vi "message_send.vi"(0 "Host_Reference":refnum<class "HGF_Reference.lvclass">, 1 "addressee":string, 2 "addressee interface":string, 3 "type":enum16{"mobile Agent", "Visitor", "Message"}(ring)=enum."Message", 4 "message":string, 5 "error in (no error)":errorcluster, 6 "request reply":bool=TRUE, 7 "message name":enum16{"travel request", "PublicKey"}(ring), 8 "timeout in ms (-1)":i32=-1, 9 "Object":refnum<class>, 11 "communication type":enum16{"SV", "Dim"}(ring)) -> (14 "dup Host_Reference":refnum<class "HGF_Reference.lvclass">, 19 "error out":errorcluster)   [LabVIEW 2009, in "MoAgSy.lvlib" / "MoAgSy_Host.lvclass"]
doc: "<B>Public</B> VI creates a new message and delivers it to addressee.\nReferenced Host is sender and will receive the reply.\n<B>still in progress\nError handling\n</B>\nF.Berck@gsi.de\nGSI Darmstadt 2009"
uses:
  MoAgSy_Host.lvclass
  HGF_BaseClasses/HGF_Reference/HGF_Reference.lvclass
  MoAgSy_Message/MoAgSy_Message.lvclass
  MoAgSy_Factory/MoAgSy_Factory.lvclass
  HGF_BaseClasses/HGF_Factory/HGF_Factory.lvclass
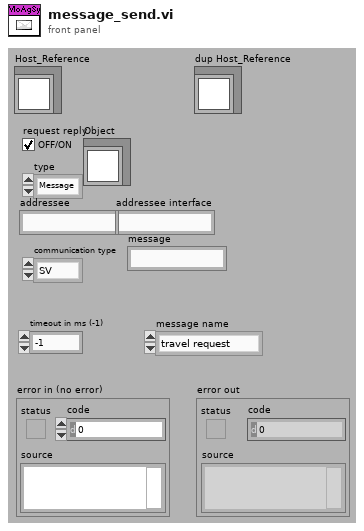
[diagram p1: front panel]
types:
  T1 = cluster{"Host Variable":refnum<k21>, "Agent_Event (Monitor Event)":refnum<class "HGF_Event.lvclass">, "Host_Event (Monitor Event)":refnum<class "HGF_Event.lvclass">, "DSCException":refnum<class "HGF_TriggeredEvent.lvclass">, "MoAgSy_DSCThreadPool":refnum<class "HGF_Reference.lvclass">, "ManagerEvent":refnum<class "HGF_Event.lvclass">, "DSCDestination":refnum<class "HGF_TriggeredEvent.lvclass">}
  T2 = cluster{"Host Name":string, "Maximum number of running Agents":i16, "ID":string}
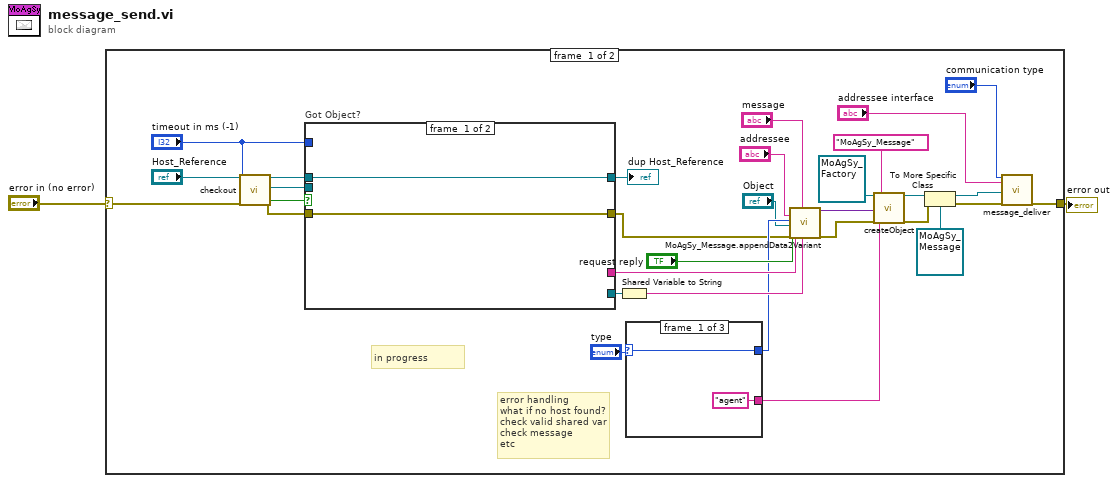
[diagram p0: block diagram]
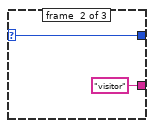
[diagram p2: hidden frame]
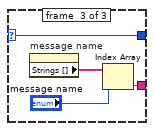
[diagram p3: hidden frame]
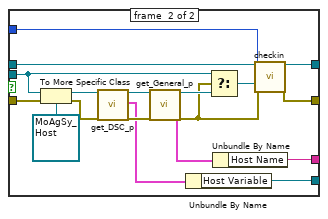
[diagram p4: hidden frame]
diagram:
  n1 = case shown="No Error" "error in (no error)" {
    selector: "error in (no error)" -> [w12 w62]
    tunnel: [w13 w62] -> w2
    frame #0 {
      # "error handling\nwhat if no host found?\ncheck valid shared var\ncheck message\netc"
      # "in progress"
      n2 = call "checkout.vi"("HGF_Reference"="Host_Reference", "timeout in ms (-1)"="timeout in ms (-1)", "error in (no error)"=w12) -> ("dup HGF_Reference"=w30:refnum<class "HGF_Reference.lvclass">, "Object"=w32:refnum<class>, "got object?"=w31:bool, "error out"=w33:errorcluster)  [unwired: 13 out]
      n3 = case "Got Object?" shown="True" w31 {
        tunnel: w32 -> [_ w54]
        tunnel: w30 -> [w43 w60]
        tunnel: [w43 w59] -> w28
        tunnel: "timeout in ms (-1)" -> [_ w58]
        tunnel: [w42 w57] -> w5
        tunnel: w33 -> [w42 w56]
        tunnel: [_ w50] -> w24
        tunnel: [_ w44] -> w15
        frame #0 {
        }
        frame #1 {
          n4 = To More Specific Class(target class=refnum<class "MoAgSy_Host.lvclass"> refnum ("MoAgSy.lvlib:MoAgSy_Host.lvclass"), reference=w54, error in=w56) -> (specific class reference=w49:refnum<class "MoAgSy_Host.lvclass">, error out=w47:errorcluster)
          n5 = call "get_DSC_p.vi"("MoAgSy_Host"=w49, "error in (no error)"=w47) -> ("dup MoAgSy_Host"=w48:refnum<class "MoAgSy_Host.lvclass">, "DSC"=w45:T1, "error out"=w46:errorcluster)  [unwired: 15 out]
          n6 = call "get_General_p.vi"("MoAgSy_Host"=w48, "error in (no error)"=w46) -> ("dup MoAgSy_Host"=w53:refnum<class "MoAgSy_Host.lvclass">, "General"=w51:T2, "error out"=w52:errorcluster)  [unwired: 15 out]
          n7 = Unbundle By Name(w45) -> ("Host Variable"=w44:refnum<k21>)
          n8 = Select(t=w54, s=w52, f=w53) -> (s? t:f=w55:refnum<class>)
          n9 = Unbundle By Name(w51) -> ("Host Name"=w50:string)
          n10 = call "checkin.vi"("HGF_Reference"=w60, "Object"=w55, "timeout /ms (-1)"=w58, "error in (no error)"=w52) -> ("dup HGF_Reference"=w59:refnum<class "HGF_Reference.lvclass">, "error out"=w57:errorcluster)  [unwired: 14 out]
        }
      }
      "dup Host_Reference" <- w28
      n11 = Shared Variable to String(1:w15) -> (0:w14:string)
      n12 = case shown="\"Message\"" "type" {
        selector: "type" -> [w35 w37 w41]
        tunnel: [w35 w37 w41] -> w9
        tunnel: ["agent" "visitor" w38] -> w8
        frame #0 {
        }
        frame #1 {
        }
        frame #2 {
          n13 = property on="message name" class="Enum (strict)"() -> ("Strings []"=w39:string[])  [unwired: 2 in, 2 out]
          n14 = Index Array(array=w39, index="message name") -> (element=w38:string)
        }
      }
      n15 = call "MoAgSy_Message.appendData2Variant.vi"("addressee"="addressee", "type"=w9, "Object"="Object", "request reply"="request reply", "error in"=w5, "sender"=w24, "message"="message", "reply to"=w14) -> ("dup_initData"=w23:variant, "error out"=w22:errorcluster)  [unwired: 3 in, 7 out]
      n16 = call "createObject.vi"("HGF_Factory"=refnum<class "MoAgSy_Factory.lvclass"> refnum ("MoAgSy.lvlib:MoAgSy_Factory.lvclass"), "objectName"=w8, "initializationData"=w23, "error in (no error)"=w22, "className"="MoAgSy_Message") -> ("HGF_Object"=w21:refnum<class "HGF_Factory.lvclass">, "error out"=w20:errorcluster)  [unwired: 13 out]
      n17 = To More Specific Class(target class=refnum<class "MoAgSy_Message.lvclass"> refnum ("MoAgSy.lvlib:MoAgSy_Message.lvclass"), reference=w21, error in=w20) -> (specific class reference=w17:refnum<class "MoAgSy_Message.lvclass">, error out=w19:errorcluster)
      n18 = call "message_deliver.vi"("communication type"="communication type", "shared variable refnum"="addressee interface", "MoAgSy_Message"=w17, "error in (no error)"=w19) -> ("error out"=w13:errorcluster)  [unwired: 15 out]
    }
    frame #1 {
    }
  }
  "error out" <- w2
